vi "Main Power Grid.vi"() -> ()   [LabVIEW 2024]
panel:
  in  "Auto Balance":bool
  out "Grid Power (KW)":dbl(knob)=97.0 scale=0.0..1000.0
  out "CO2 Accumulation":i32(graph)
  out "Load Balance":dbl(knob)=-103.0 scale=-500.0..500.0
  out "Loads Requested":dbl(knob)=200.0 scale=0.0..1000.0
  out "Kilowatts Generated":T1(graph)={"Array[0]"=0.01, "Array[1]"=-200.0, "Array[2]"=97.0, "Array[3]"=0.0, "Array[4]"=0.0, "Array[5]"=0.0, "Array[6]"=0.0, "Array[7]"=0.0, "Array[8]"=0.0}
  out "All Values":dbl[][](array[numeric])=[[705.0, 0.01, 100.0, 0.0, 0.0, 0.0, 8.4], [-800.0, -200.0, -200.0, 0.0, 0.0, -1.0, 120.0], [290.0, 97.0, 0.0, 97.0, 0.0, 1.0, 95.0], [0.0, 0.0, 0.0, 0.0, 0.0, -1.0, 0.0], [290.0, 0.0, 0.0, 0.0, 0.0, 1.0, 0.0]] format="%_3f"
  out "Values Read":dbl[][](array[numeric]) format="%_3g"
  out "USB Device Address":string[](array[string])=["ASRL15::INSTR", "ASRL16::INSTR", "ASRL17::INSTR", "ASRL18::INSTR", "ASRL19::INSTR"]
  in  "stop":bool
  in  "Send  Cmd":bool[](array[boolean])=[FALSE, FALSE, FALSE, FALSE, FALSE]
  in  "Parameters to Send (input)":dbl[][](array[numeric])=[[0.0, 0.0, 0.0, 0.0], [0.0, 0.0, 0.0, 0.0], [0.0, 0.0, 0.0, 0.0], [0.0, 0.0, 0.0, 0.0], [0.0, 0.0, 0.0, 0.0]]
  in  "Ring 10":u16(ring)
  in  "Ring 9":u16(ring)
  in  "Ring 8":u16(ring)
  in  "Ring 7":u16(ring)
  in  "Ring 6":u16(ring)
  in  "Ring 5":u16(ring)
  in  "Ring 4":u16(ring)
  in  "Ring 3":u16(ring)
  in  "Ring 2":u16(ring)
  in  "Ring":u16(ring)
  out "System":string[](array[string])=["generator\r\n", "houseload\r\n", "solartracker\r\n", "fan\r\n", "windturbine\r\n"]
  # "KW Gen"
  # "KW Cap"
  # "KW Load"
  # "KW Balance"
  # "CO2 Emis"
  # "Line Voltage"
  # "Device Commands"
  # "Renewable"
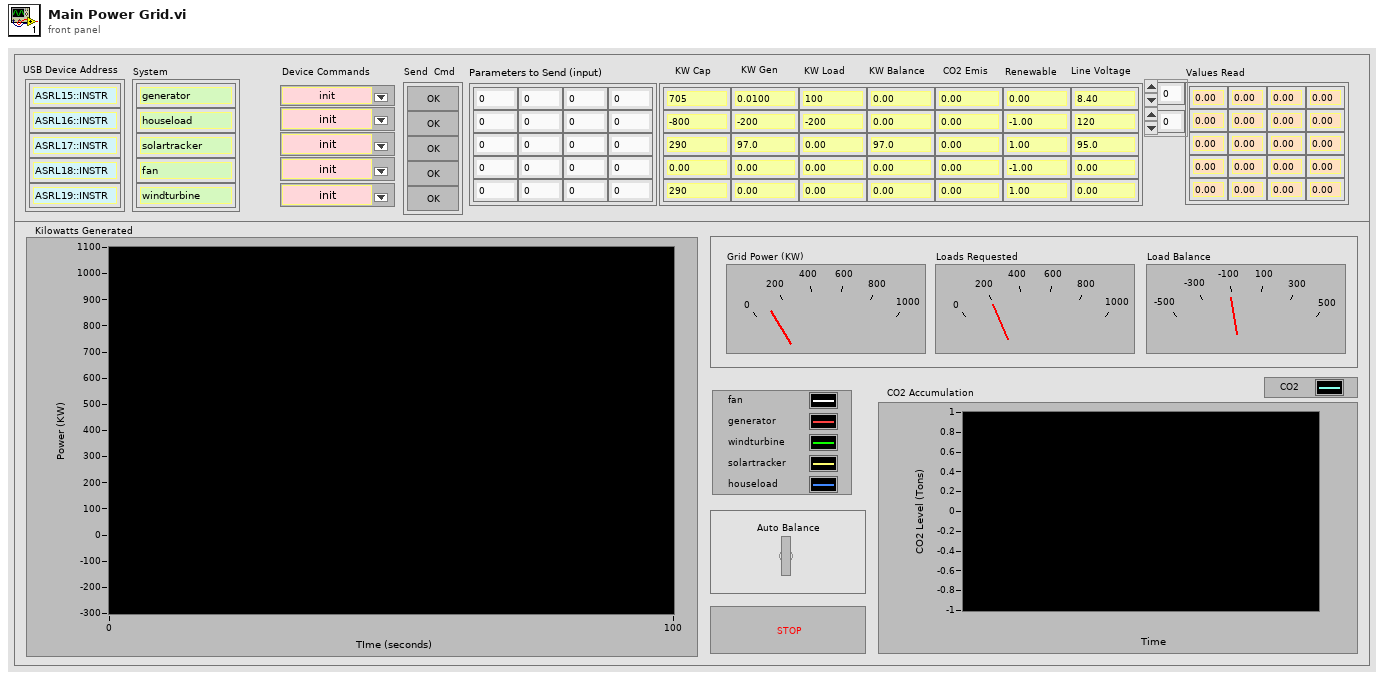
[diagram p1: front panel]
types:
  T1 = cluster{"Array[0]":dbl, "Array[1]":dbl, "Array[2]":dbl, "Array[3]":dbl, "Array[4]":dbl, "Array[5]":dbl, "Array[6]":dbl, "Array[7]":dbl, "Array[8]":dbl}
  T2 = cluster{"Array[0]":i32, "Array[1]":i32, "Array[2]":i32, "Array[3]":i32, "Array[4]":i32, "Array[5]":i32, "Array[6]":i32, "Array[7]":i32, "Array[8]":i32}[]
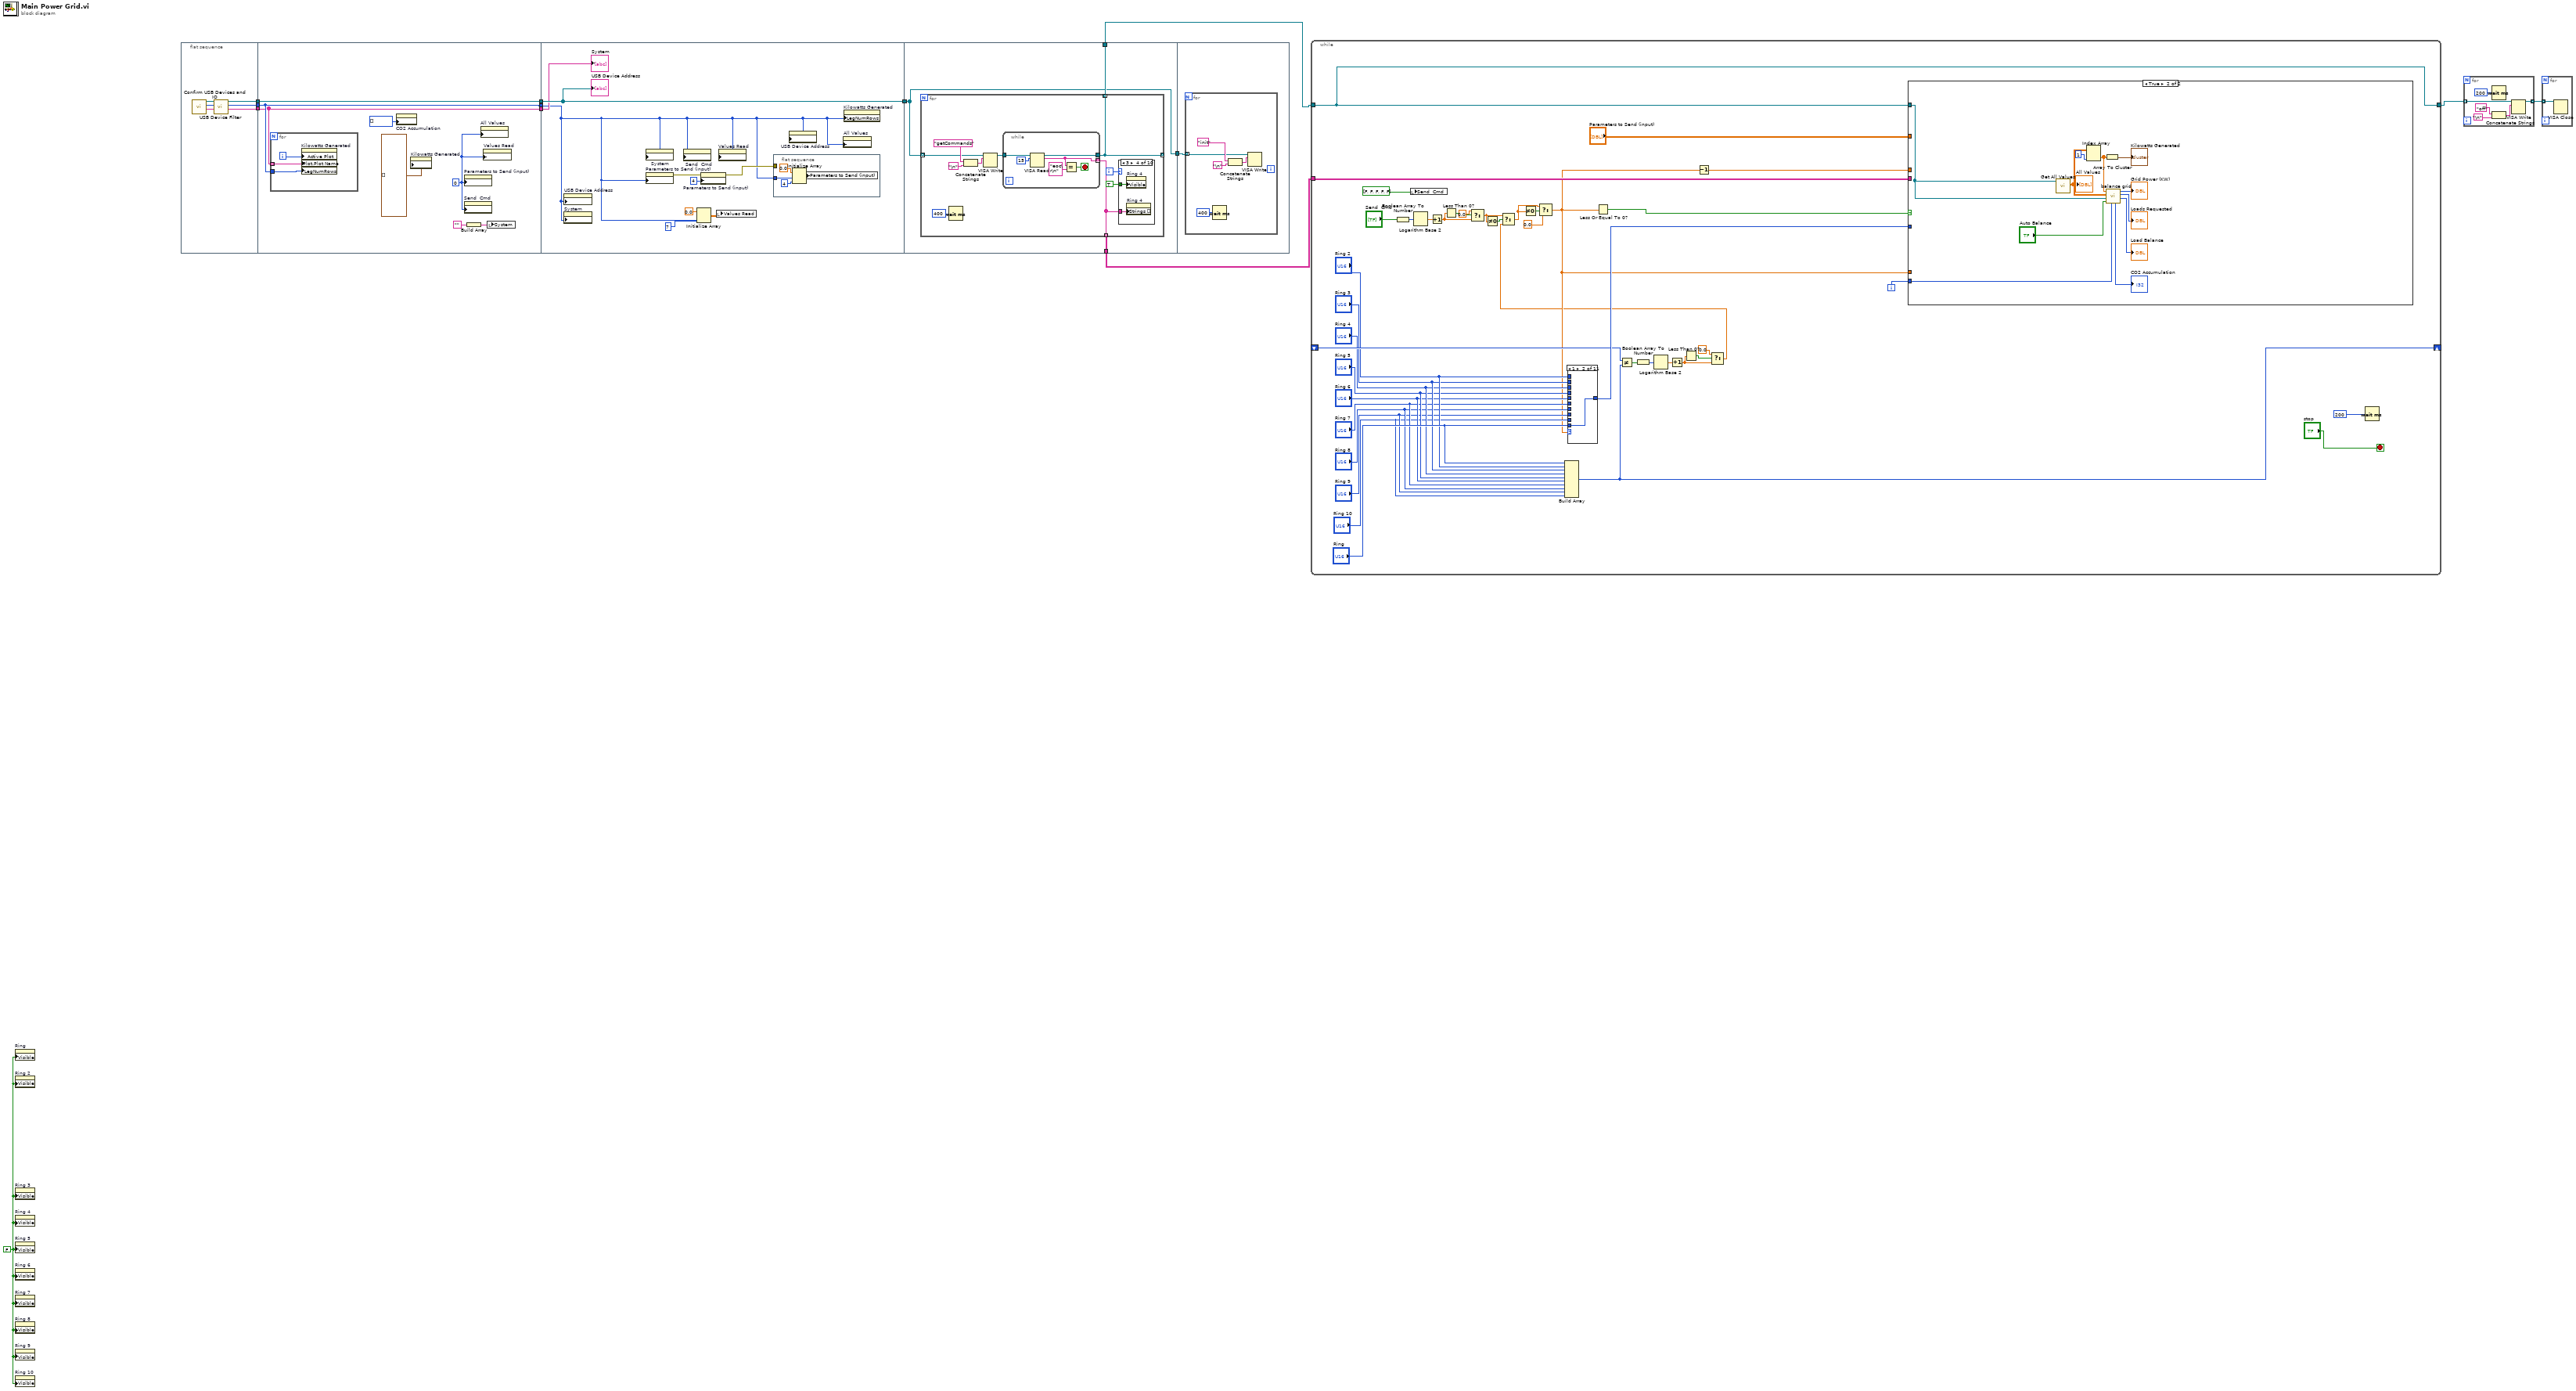
[diagram p0: block diagram]
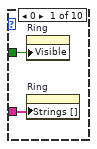
[diagram p2: hidden frame]
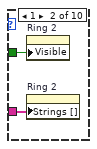
[diagram p3: hidden frame]
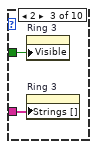
[diagram p4: hidden frame]
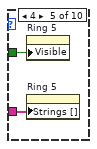
[diagram p5: hidden frame]
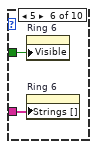
[diagram p6: hidden frame]
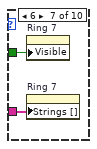
[diagram p7: hidden frame]
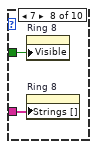
[diagram p8: hidden frame]
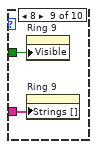
[diagram p9: hidden frame]
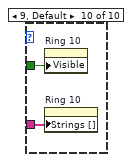
[diagram p10: hidden frame]
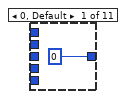
[diagram p11: hidden frame]
diagram:
  w13 = FALSE ("Visible")
  n1 = property on="Ring" class="Ring (strict)"("Visible"=w13) -> ()  [unwired: 2 in, 2 out]
  n2 = property on="Ring 2" class="Ring (strict)"("Visible"=w13) -> ()  [unwired: 2 in, 2 out]
  n3 = property on="Ring 3" class="Ring (strict)"("Visible"=w13) -> ()  [unwired: 2 in, 2 out]
  n4 = property on="Ring 4" class="Ring (strict)"("Visible"=w13) -> ()  [unwired: 2 in, 2 out]
  n5 = property on="Ring 5" class="Ring (strict)"("Visible"=w13) -> ()  [unwired: 2 in, 2 out]
  n6 = property on="Ring 6" class="Ring (strict)"("Visible"=w13) -> ()  [unwired: 2 in, 2 out]
  n7 = property on="Ring 7" class="Ring (strict)"("Visible"=w13) -> ()  [unwired: 2 in, 2 out]
  n8 = property on="Ring 8" class="Ring (strict)"("Visible"=w13) -> ()  [unwired: 2 in, 2 out]
  n9 = property on="Ring 9" class="Ring (strict)"("Visible"=w13) -> ()  [unwired: 2 in, 2 out]
  n10 = property on="Ring 10" class="Ring (strict)"("Visible"=w13) -> ()  [unwired: 2 in, 2 out]
  n11 = flat-sequence {
    tunnel: [w16] -> w4
    tunnel: [w15] -> w3
    tunnel: [w14] -> w2
    tunnel: w4 -> [w22]
    tunnel: w3 -> [w21]
    tunnel: w2 -> [w20]
    tunnel: [w22] -> w10
    tunnel: [w20] -> w9
    tunnel: [w21] -> w8
    tunnel: w10 -> [w39]
    tunnel: w9 -> [w32]
    tunnel: w8 -> [w31]
    tunnel: [w39] -> w7
    tunnel: w7 -> [w44]
    tunnel: [w46] -> w6
    tunnel: [w45] -> w5
    tunnel: [w44] -> w1
    tunnel: w1 -> [w83]
    frame #0 {
      n12 = call "Confirm USB Devices and IO.vi"() -> ("Device Name"=w19:string[], "Num Dev"=w18:u32, "Device Address"=w17:refnum<visa-resource-name>[])  [unwired: 9 in]
      n13 = call "USB Device Filter.vi"("Device Name"=w19, "Num Dev"=w18, "Device Address"=w17) -> ("Device Name 2"=w14:string[], "Num Dev 2"=w15:u32, "Device Address 2"=w16:refnum<visa-resource-name>[])  [unwired: 6 in]
    }
    frame #1 {
      w25 = 0
      n14 = for {
        tunnel: w21 -> [w29]
        tunnel: w20 -> [w28] mode=indexing
        i -> [w30]
        n15 = property on="Kilowatts Generated" class="WFChart (strict)"("Active Plot"=w30, "Plot.Plot Name"=w28, "LegNumRows"=w29) -> ()  [unwired: 2 in, 2 out]
      }
      n16 = property on="CO2 Accumulation" class="WFChart (strict)"("History Data"=i32[] []) -> ()  [unwired: 2 in, 2 out]
      n17 = property on="Kilowatts Generated" class="WFChart (strict)"("History Data"=T2 []) -> ()  [unwired: 2 in, 2 out]
      n18 = property on="Parameters to Send (input)" class="Arr (strict)"("Number of Rows"=w25) -> ()  [unwired: 2 in, 2 out]
      n19 = property on="Send  Cmd" class="Arr"("Number of Rows"=w25) -> ()  [unwired: 2 in, 2 out]
      n20 = Build Array("") -> (w26:string[])
      n21 = property on="All Values" class="Arr (strict)"("Number of Rows"=w25) -> ()  [unwired: 2 in, 2 out]
      n22 = property on="Values Read" class="Arr (strict)"("Number of Rows"=w25) -> ()  [unwired: 2 in, 2 out]
      n23 = local write "System"(w26) -> ()
    }
    frame #2 {
      n24 = property on="USB Device Address" class="Arr (strict)"("Number of Rows"=w31) -> ()  [unwired: 2 in, 2 out]
      n25 = property on="System" class="Arr (strict)"("Number of Rows"=w31) -> ()  [unwired: 2 in, 2 out]
      n26 = property on="System" class="Arr (strict)"("Number of Rows"=w31) -> ()  [unwired: 2 in, 2 out]
      n27 = property on="Parameters to Send (input)" class="Arr (strict)"("Number of Rows"=w31) -> (error out=w36:errorcluster)  [unwired: 2 in, 1 out]
      n28 = property on="Send  Cmd" class="Arr"("Number of Rows"=w31) -> ()  [unwired: 2 in, 2 out]
      n29 = Initialize Array(0.0 ("element"), w31, 7 ("dimension size")) -> (w37:dbl[][])
      n30 = property on="Parameters to Send (input)" class="Arr (strict)"(error in=w36, "Number of Columns"=u32 4) -> (error out=w38:errorcluster)  [unwired: 1 in, 1 out]
      n31 = local write "Values Read"(w37) -> ()
      n32 = property on="Values Read" class="Arr (strict)"("Number of Rows"=w31) -> ()  [unwired: 2 in, 2 out]
      n33 = flat-sequence {
        tunnel: w38 -> [_]
        tunnel: w31 -> [w41]
        frame #0 {
          n34 = Initialize Array(0.0 ("element"), w41, 4 ("dimension size")) -> (w42:dbl[][])
          n35 = local write "Parameters to Send (input)"(w42) -> ()
        }
      }
      n36 = property on="USB Device Address" class="Arr (strict)"("Number of Rows"=w31) -> ()  [unwired: 2 in, 2 out]
      n37 = property on="All Values" class="Arr (strict)"("Number of Rows"=w31) -> ()  [unwired: 2 in, 2 out]
      n38 = property on="Kilowatts Generated" class="WFChart (strict)"("LegNumRows"=w31) -> ()  [unwired: 2 in, 2 out]
      "System" <- w32
      "USB Device Address" <- w39
    }
    frame #3 {
      n39 = for {
        tunnel: [w47] -> _ mode=indexing
        tunnel: w44 -> [w52] mode=indexing
        tunnel: [w48] -> w46 mode=indexing
        tunnel: [w47] -> w45 mode=indexing
        i -> [w51]
        n40 = Wait (ms)(milliseconds to wait=u32 400) -> ()  [unwired: 1 out]
        n41 = Concatenate Strings("getCommands", "\n") -> (w55:string)
        n42 = VISA Write(VISA resource name=w52, write buffer=w55) -> (VISA resource name out=w53:refnum<visa-resource-name>)  [unwired: 1 in, 2 out]
        n43 = while {
          tunnel: [w78] -> w48 mode=indexing
          tunnel: [w80] -> w47
          tunnel: w53 -> [w79]
          stop <- w81 stop-if-true
          n44 = VISA Read(VISA resource name=w79, byte count=u32 15) -> (VISA resource name out=w80:refnum<visa-resource-name>, read buffer=w78:string)  [unwired: 1 in, 2 out]
          n45 = Equal?(x=w78, y="eoc\r\n" ("read buffer")) -> (x = y?=w81:bool)
        }
        n46 = case shown="3" w51 {
          tunnel: w48 -> [w58 w60 w62 w64 w66 w68 w70 w72 w74 w76]
          tunnel: TRUE -> [w57 w59 w61 w63 w65 w67 w69 w71 w73 w75]
          frame 0 {
            n47 = property on="Ring" class="Ring (strict)"("Visible"=w57) -> ()  [unwired: 2 in, 2 out]
            n48 = property on="Ring" class="Ring (strict)"("Strings []"=w58) -> ()  [unwired: 2 in, 2 out]
          }
          frame 1 {
            n49 = property on="Ring 2" class="Ring (strict)"("Visible"=w59) -> ()  [unwired: 2 in, 2 out]
            n50 = property on="Ring 2" class="Ring (strict)"("Strings []"=w60) -> ()  [unwired: 2 in, 2 out]
          }
          frame 2 {
            n51 = property on="Ring 3" class="Ring (strict)"("Visible"=w61) -> ()  [unwired: 2 in, 2 out]
            n52 = property on="Ring 3" class="Ring (strict)"("Strings []"=w62) -> ()  [unwired: 2 in, 2 out]
          }
          frame 3 {
            n53 = property on="Ring 4" class="Ring (strict)"("Visible"=w63) -> ()  [unwired: 2 in, 2 out]
            n54 = property on="Ring 4" class="Ring (strict)"("Strings []"=w64) -> ()  [unwired: 2 in, 2 out]
          }
          frame 4 {
            n55 = property on="Ring 5" class="Ring (strict)"("Visible"=w65) -> ()  [unwired: 2 in, 2 out]
            n56 = property on="Ring 5" class="Ring (strict)"("Strings []"=w66) -> ()  [unwired: 2 in, 2 out]
          }
          frame 5 {
            n57 = property on="Ring 6" class="Ring (strict)"("Visible"=w67) -> ()  [unwired: 2 in, 2 out]
            n58 = property on="Ring 6" class="Ring (strict)"("Strings []"=w68) -> ()  [unwired: 2 in, 2 out]
          }
          frame 6 {
            n59 = property on="Ring 7" class="Ring (strict)"("Visible"=w69) -> ()  [unwired: 2 in, 2 out]
            n60 = property on="Ring 7" class="Ring (strict)"("Strings []"=w70) -> ()  [unwired: 2 in, 2 out]
          }
          frame 7 {
            n61 = property on="Ring 8" class="Ring (strict)"("Visible"=w71) -> ()  [unwired: 2 in, 2 out]
            n62 = property on="Ring 8" class="Ring (strict)"("Strings []"=w72) -> ()  [unwired: 2 in, 2 out]
          }
          frame 8 {
            n63 = property on="Ring 9" class="Ring (strict)"("Visible"=w73) -> ()  [unwired: 2 in, 2 out]
            n64 = property on="Ring 9" class="Ring (strict)"("Strings []"=w74) -> ()  [unwired: 2 in, 2 out]
          }
          frame 9, Default {
            n65 = property on="Ring 10" class="Ring (strict)"("Visible"=w75) -> ()  [unwired: 2 in, 2 out]
            n66 = property on="Ring 10" class="Ring (strict)"("Strings []"=w76) -> ()  [unwired: 2 in, 2 out]
          }
        }
      }
    }
    frame #4 {
      n67 = for {
        tunnel: w83 -> [w85] mode=indexing
        n68 = Wait (ms)(milliseconds to wait=u32 400) -> ()  [unwired: 1 out]
        n69 = Concatenate Strings("init", "\n") -> (w87:string)
        n70 = VISA Write(VISA resource name=w85, write buffer=w87) -> ()  [unwired: 1 in, 3 out]
      }
    }
  }
  n71 = while {
    tunnel: [w119] -> w12
    tunnel: w5 -> [w119]
    tunnel: w6 -> [w124]
    shift-right: [w117] -> _
    shift-left: _ -> [w116]
    i -> [w120]
    stop <- "stop" stop-if-true
    n72 = Boolean Array To Number(Boolean array="Send  Cmd") -> (number=w128:u32)
    n73 = local write "Send  Cmd"(bool[] [FALSE, FALSE, FALSE, FALSE, FALSE] ("Send Command")) -> ()
    n74 = Logarithm Base 2(1:w128) -> (0:w127:dbl)
    n75 = Increment(x=w127) -> (x+1=w103:dbl)
    n76 = Less Than 0?(x=w103) -> (x < 0?=w104:bool)
    n77 = Select(t=0.0, s=w104, f=w103) -> (s? t:f=w89:dbl)
    n78 = Not Equal To 0?(x=w89) -> (x != 0?=w101:bool)
    n79 = Build Array("Ring", "Ring 2", "Ring 3", "Ring 4", "Ring 5", "Ring 6", "Ring 7", "Ring 8", "Ring 9", "Ring 10") -> (w117:u16[])
    n80 = Not Equal?(x=w116, y=w117) -> (x != y?=w96:bool[])
    n81 = Boolean Array To Number(Boolean array=w96) -> (number=w91:u32)
    n82 = Logarithm Base 2(1:w91) -> (0:w95:dbl)
    n83 = Increment(x=w95) -> (x+1=w93:dbl)
    n84 = Less Than 0?(x=w93) -> (x < 0?=w94:bool)
    n85 = Select(t=0.0, s=w94, f=w93) -> (s? t:f=w90:dbl)
    n86 = Select(t=w89, s=w101, f=w90) -> (s? t:f=w100:dbl)
    n87 = Not Equal To 0?(x=w100) -> (x != 0?=w99:bool)
    n88 = Select(t=w100, s=w99, f=0.0) -> (s? t:f=w97:dbl)
    n89 = case shown="1" w97 {
      tunnel: "Ring" -> [_ w131 _ _ _ _ _ _ _ _ _]
      tunnel: [u16 0 ("Ring 10") w131 w132 w133 w134 w135 w136 w137 w138 w139 w140] -> w118
      tunnel: "Ring 2" -> [_ _ w132 _ _ _ _ _ _ _ _]
      tunnel: "Ring 3" -> [_ _ _ w133 _ _ _ _ _ _ _]
      tunnel: "Ring 4" -> [_ _ _ _ w134 _ _ _ _ _ _]
      tunnel: "Ring 5" -> [_ _ _ _ _ w135 _ _ _ _ _]
      tunnel: "Ring 6" -> [_ _ _ _ _ _ w136 _ _ _ _]
      tunnel: "Ring 7" -> [_ _ _ _ _ _ _ w137 _ _ _]
      tunnel: "Ring 8" -> [_ _ _ _ _ _ _ _ w138 _ _]
      tunnel: "Ring 9" -> [_ _ _ _ _ _ _ _ _ w139 _]
      tunnel: "Ring 10" -> [_ _ _ _ _ _ _ _ _ _ w140]
      frame 0, Default {
      }
      frame 1 {
      }
      frame 2 {
      }
      frame 3 {
      }
      frame 4 {
      }
      frame 5 {
      }
      frame 6 {
      }
      frame 7 {
      }
      frame 8 {
      }
      frame 9 {
      }
      frame 10 {
      }
    }
    n90 = Less Or Equal To 0?(x=w97) -> (x <= 0?=w115:bool)
    n91 = Decrement(x=w97) -> (x-1=w122:dbl)
    n92 = case shown="True" w115 {
      tunnel: w124 -> [w148 _]
      tunnel: w119 -> [w145 w187]
      tunnel: w122 -> [w147 _]
      tunnel: "Parameters to Send (input)" -> [w146 _]
      tunnel: w97 -> [w143 _]
      tunnel: w118 -> [w144 _]
      tunnel: w120 -> [_ w186]
      frame False {
        n93 = Index Array(array=w148, index (row)=w147, index (col)=w144) -> (element=w154:string)
        n94 = Index Array(array=w146, index (row)=w147) -> (element=w156:dbl[])  [unwired: 1 in]
        n95 = Search/Split String(string=w154, search string/char (-)="\n") -> (substring before match=w141:string)  [unwired: 1 in, 2 out]
        n96 = Index Array(array=w145, index=w147) -> (element=w155:refnum<visa-resource-name>)
        n97 = String Length(string=w141) -> (length=w151:i32)
        n98 = Decrement(x=w151) -> (x-1=w152:i32)
        n99 = Decrement(x=w152) -> (x-1=w153:i32)
        n100 = String Subset(string=w141, offset (0)=w153, length (rest)=1 ("length (rest)")) -> (substring=w150:string)
        n101 = case shown="\">\"" w150 {
          tunnel: w141 -> [w157 w162 w184]
          tunnel: w155 -> [w158 w163 w183]
          tunnel: w156 -> [_ w161 _]
          tunnel: w143 -> [_ _ w181]
          frame "False", Default {
            n102 = Concatenate Strings(w157, "\n") -> (w159:string)
            n103 = VISA Write(VISA resource name=w158, write buffer=w159) -> ()  [unwired: 1 in, 3 out]
          }
          frame ">" {
            n104 = Search/Split String(string=w162, search string/char (-)=">") -> (substring before match=w165:string, match + rest of string=w168:string)  [unwired: 1 in, 1 out]
            n105 = String Subset(string=w168, offset (0)=1, length (rest)=1 ("length (rest)")) -> (substring=w170:string)
            n106 = Concatenate Strings(w165, "\n") -> (w164:string)
            n107 = Decimal String To Number(string=w170) -> (number=w169:i32)  [unwired: 2 in, 1 out]
            n108 = VISA Write(VISA resource name=w163, write buffer=w164) -> (VISA resource name out=w166:refnum<visa-resource-name>)  [unwired: 1 in, 2 out]
            n109 = for {
              N: w169 -> [_]
              tunnel: w166 -> [w178]
              tunnel: w161 -> [w177] mode=indexing
              n110 = Number To Decimal String(number=w177) -> (decimal integer string=w175:string)  [unwired: 1 in]
              n111 = Wait (ms)(milliseconds to wait=u32 100) -> ()  [unwired: 1 out]
              n112 = Concatenate Strings(w175, "\n") -> (w174:string)
              n113 = VISA Write(VISA resource name=w178, write buffer=w174) -> ()  [unwired: 1 in, 3 out]
            }
          }
          frame "<" {
            n114 = local read "Values Read"() -> (w180:dbl[][])
            n115 = call "Command with Return Value.vi"("y"=w181, "read buffer"=w184, "Values Read in"=w180, "VISA Refnum in"=w183) -> ("Values Read out"=→"Values Read":dbl[][])  [unwired: 7 in]
          }
        }
      }
      frame True {
        n116 = call "Get All Values.vi"("Array 2"=w187) -> ("Array"=w193:dbl[][])  [unwired: 9 in, 1 out]
        "All Values" <- w193
        n117 = Index Array(array=w193, index (col)=1 ("disabled index (col)")) -> (element=w189:dbl[])  [unwired: 1 in]
        n118 = Array To Cluster(array=w189) -> (cluster=→"Kilowatts Generated":T1)
        n119 = call "balance grid.vi"("init(0)"=w186, "Balance"="Auto Balance", "Device Addresses"=w187, "All Values"=w193, "KW Values"=w189) -> ("Load Balance"=→"Load Balance":i32, "Loads Requested"=→"Loads Requested":i32, "Grid Power (KW)"=→"Grid Power (KW)":i32, "CO2 Accum"=→"CO2 Accumulation":i32)  [unwired: 3 in]
      }
    }
    n120 = Wait (ms)(milliseconds to wait=u32 200) -> ()  [unwired: 1 out]
  }
  n121 = for {
    tunnel: w12 -> [w201] mode=indexing
    tunnel: [w200] -> w11 mode=indexing
    n122 = Wait (ms)(milliseconds to wait=u32 200) -> ()  [unwired: 1 out]
    n123 = Concatenate Strings("off" ("string"), "\n") -> (w197:string)
    n124 = VISA Write(VISA resource name=w201, write buffer=w197) -> (VISA resource name out=w200:refnum<visa-resource-name>)  [unwired: 1 in, 2 out]
  }
  n125 = for {
    tunnel: w11 -> [w202] mode=indexing
    n126 = VISA Close(VISA resource name=w202) -> ()  [unwired: 1 in, 1 out]
  }
